vi "Read Error Pointer.vi"(8 "error in (no error)":errorcluster, 11 "Thread in":refnum<class "Thread.lvclass">) -> (0 "error out":errorcluster, 2 "error":errorcluster, 3 "Thread out":refnum<class "Thread.lvclass">)   [LabVIEW 2017, in "DSF Core.lvlib" / "Thread.lvclass"]
uses:
  Thread.lvclass
  Thread.lvclass/Thread.ctl
  Pointers/Error/Error Pointer.lvclass
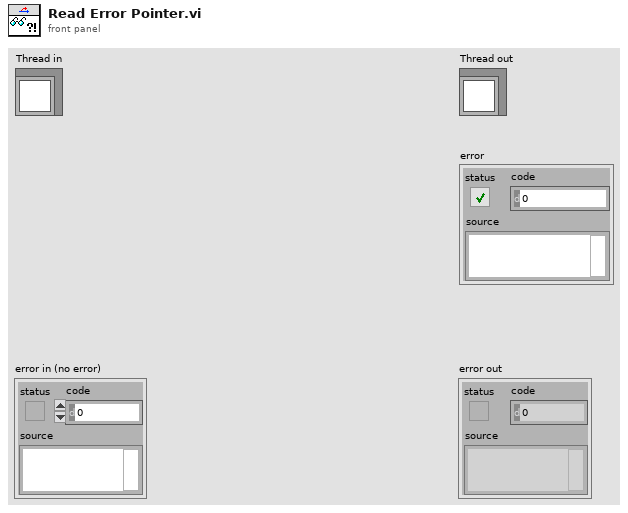
[diagram p1: front panel]
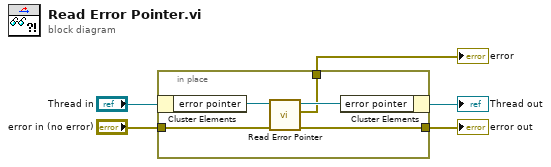
[diagram p0: block diagram]
diagram:
  n1 = in-place {
    in-place-border: [w8] -> w4
    in-place-border: "error in (no error)" -> [w10]
    in-place-border: [w6] -> w1
    n2 = in-place-cluster #1("Thread in") -> ("error pointer"=w9:refnum<class "Error Pointer.lvclass">)
    n3 = call "Read Error Pointer.vi"("error in (no error)"=w10, "Error Pointer in"=w9) -> ("error out"=w8:errorcluster, "error"=w6:errorcluster, "Error Pointer in"=w7:refnum<class "Error Pointer.lvclass">)  [unwired: 7 in]
    n4 = in-place-cluster #1("error pointer"=w7) -> (→"Thread out":refnum<class "Thread.lvclass">)
  }
  "error out" <- w4
  "error" <- w1
